vi "WPI_IMU_ADIS16460_HardwareResetDelay.vi"(7 "Delay (ms)":dbl=5000.0 format="%#_13g", 8 "error in":errorcluster, 11 "DigitalOutputDevRef":T1={"DIO Channel"=enum."DIO 1", "DevStatus"={"status"=FALSE, "code"=0, "source"=""}}) -> (0 "error out":errorcluster, 3 "DigitalOutputDevRef":T1={"DIO Channel"=enum."DIO 1", "DevStatus"={"status"=FALSE, "code"=0, "source"=""}})   [LabVIEW 2015, in "FRC ADIS16460.lvlib"]
uses:
  <vilib>/Rock Robotics/WPI/DigitalOutput/WPI_DigitalOutputDevRef.ctl
  <vilib>/Rock Robotics/SystemInterfaces/DIO/FPGA_DIOChannel.ctl
  FRC ADIS16460.lvlib
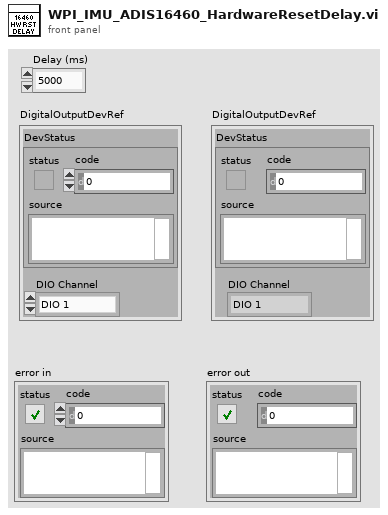
[diagram p1: front panel]
types:
  T1 = typedef "WPI_DigitalOutputDevRef.ctl" = cluster{"DIO Channel":T2, "DevStatus":errorcluster}
  T2 = typedef "FPGA_DIOChannel.ctl" = enum8{"DIO 0", "DIO 1", "DIO 2", "DIO 3", "DIO 4", "DIO 5", "DIO 6", "DIO 7", "DIO 8", "DIO 9", "DIO MXP 0", "DIO MXP 1", "DIO MXP 2", "DIO MXP 3", "DIO MXP 4", "DIO MXP 5", "DIO MXP 6", "DIO MXP 7", "DIO MXP 8", "DIO MXP 9", "DIO MXP 10", "DIO MXP 11", "DIO MXP 12", "DIO MXP 13", "DIO MXP 14", "DIO MXP 15", "Invalid"}
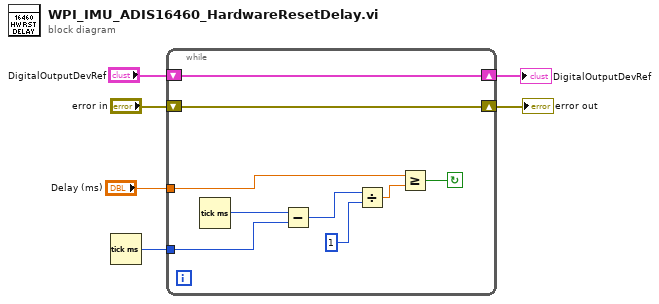
[diagram p0: block diagram]
diagram:
  n1 = Tick Count (ms)() -> (millisecond timer value=w6:u32)
  n2 = while {
    tunnel: "Delay (ms)" -> [w8]
    tunnel: w6 -> [w12]
    shift-right: [w15] -> w3
    shift-left: "error in" -> [w15]
    shift-right: [w14] -> w1
    shift-left: "DigitalOutputDevRef" -> [w14]
    stop <- w7 continue-if-true
    n3 = Tick Count (ms)() -> (millisecond timer value=w13:u32)
    n4 = Subtract(x=w13, y=w12) -> (x-y=w11:u32)
    n5 = Divide(x=w11, y=u32 1) -> (x/y=w9:dbl)
    n6 = Greater Or Equal?(x=w8, y=w9) -> (x >= y?=w7:bool)
  }
  "error out" <- w3
  "DigitalOutputDevRef" <- w1
